vi "SPD.Set Meas Grid.vi"(8 "Error In":errorcluster, 9 "HV_GridParams":T1, 10 "SPD.DCR Meas Setup":T15={"Strobe_code"={"Start"=0.0, "Stop"=0.0, "Step"=0.0}, "Temperature"={"Start"=-45.0, "Stop"=-45.0, "Step"=2.5}} caption="Настройка Измерений", 11 "SPD.Stand Ctrl in":T2 {"spdDeviceSession"."hidSPD.Sturtup Values"."HV_bias" format="%#_6p, V"; "spdDeviceSession"."hidSPD.Sturtup Values"."TSet" format="%#_6p, DegC"; "spdDeviceSession"."hidSPD.Controller"."HV_bias" format="%#_6p, V"; "spdDeviceSession"."hidSPD.Controller"."TSet" format="%#_6p, DegC"}) -> (0 "Error Out":errorcluster, 3 "SPD.Stand Ctrl out":T2 {"spdDeviceSession"."hidSPD.Sturtup Values"."HV_bias" format="%#_6p, V"; "spdDeviceSession"."hidSPD.Sturtup Values"."TSet" format="%#_6p, DegC"; "spdDeviceSession"."hidSPD.Controller"."HV_bias" format="%#_6p, V"; "spdDeviceSession"."hidSPD.Controller"."TSet" format="%#_6p, DegC"})   [LabVIEW 2018]
uses:
  typedefs/SPD.Grid Meas Setup.ctl
  typedefs/SPD.Test Range.ctl
  typedefs/SPD.Stand Ctrl.ctl
  Instruments/SPD HID Interface/hidSPDLibForLabView/LibVIs/hidSPD Controls/hidSPD Device Session.ctl
  Instruments/SPD HID Interface/hidSPDLibForLabView/LibVIs/hidSPD Controls/hidSPD Controller.ctl
  Instruments/SPD HID Interface/hidSPDLibForLabView/LibVIs/hidSPD Controls/hidSPD SPD Type.ctl
  Instruments/KC705 DevBoard/typedefs/DevB.Session.ctl
  Instruments/KeySight 53230A/typedefs/FreqC.Session.ctl
  Instruments/KeySight 8164B/KeySight 8164B LAN InstrLib/typedefs/KeySight 8164B control.ctl
  Instruments/LeCroy SDA830/typedefs/LeCroy.Session.ctl
  typedefs/SPD.Events.ctl
  ConfigFile/SPD.Config File ctrl.ctl
  <vilib>/Utility/config.llb/Config Data RefNum.ctl
  typedefs/SPD.Meas Result.ctl
  typedefs/SPD.Queues.ctl
  typedefs/SPD.Stand state.ctl
  MeasGrid/typedefs/SPD.HV_Grid Test Params.ctl
  <vilib>/Analysis/1siggen.llb/Ramp Pattern by Delta.vi
  <vilib>/Analysis/NI_AALBase.lvlib
  Instruments/KeySight 8164B/KeySight 8164B LAN InstrLib.lvlib
  <vilib>/Utility/config.llb/NI_LVConfig.lvlib
  Instruments/SPD HID Interface/hidSPDLibForLabView/hidSPDLibForLabView.lvlib
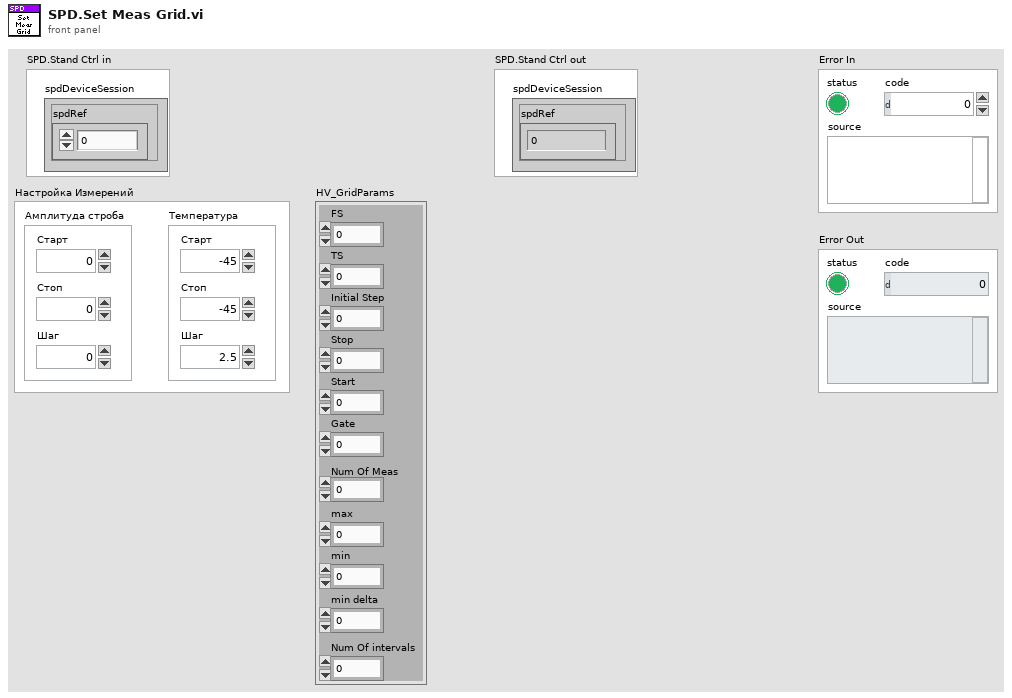
[diagram p1: front panel]
types:
  T1 = typedef "SPD.HV_Grid Test Params.ctl" = cluster{"FS":i32, "TS":i32, "Initial Step":dbl, "Stop":dbl, "Start":dbl, "Gate":dbl, "Num Of Meas":i32, "max":dbl, "min":dbl, "min delta":dbl, "Num Of intervals":i32}
  T2 = typedef "SPD.Stand Ctrl.ctl" = cluster{"spdDeviceSession":T3, "DevBSession":T6, "FreqCSession":T7, "8164BSession":T8, "LeCroySession":T9, "Events":T10, "configFile":T11, "SPD.Result":T13, "SPD.Queues":T14, "Console":refnum<vi>}
  T3 = typedef "hidSPDLibForLabView.lvlib/hidSPD Device Session.ctl" = cluster{"spdRef":u64, "connected":bool, "spdName":string, "hidSPD.Controller":T4, "hidSPD.Sturtup Values":T4, "SPD Type":T5}
  T4 = typedef "hidSPDLibForLabView.lvlib/hidSPD Controller.ctl" = cluster{"TSet":sgl, "HV_bias":sgl, "DDS_stb_code":u16}
  T5 = typedef "hidSPDLibForLabView.lvlib/hidSPD SPD Type.ctl" = enum16{"Free Run", "Gate"}
  T6 = typedef "DevB.Session.ctl" = cluster{"DevBRef":refnum<visa-resource-name>, "connected":bool}
  T7 = typedef "FreqC.Session.ctl" = cluster{"FreqCRef":refnum<visa-resource-name>, "timeout":dbl, "Gate":dbl, "connected":bool}
  T8 = typedef "KeySight 8164B LAN InstrLib.lvlib/KeySight 8164B control.ctl" = cluster{"Connection ID":refnum<k5>, "Connected":bool, "Info":string, "Slots Info":string[]}
  T9 = typedef "LeCroy.Session.ctl" = cluster{"LeCroySession":refnum<visa-resource-name>, "connected":bool}
  T10 = typedef "SPD.Events.ctl" = cluster{"DCRTest":refnum<user-event>, "Stop":refnum<user-event>}
  T11 = typedef "SPD.Config File ctrl.ctl" = cluster{"configFile ref":T12, "configFile path":path, "equipmentFile ref":T12}
  T12 = typedef "NI_LVConfig.lvlib/Config Data RefNum.ctl" = refnum<k1>
  T13 = typedef "SPD.Meas Result.ctl" = cluster{"HV_Bias":dbl[][][], "Stb_code":dbl[], "Temprature":dbl[], "Data":dbl[][][][], "DateTime":string}
  T14 = typedef "SPD.Queues.ctl" = cluster{"state queue":refnum<queue>}
  T15 = typedef "SPD.Grid Meas Setup.ctl" = cluster{"Strobe_code":T16, "Temperature":T16}
  T16 = typedef "SPD.Test Range.ctl" = cluster{"Start":dbl, "Stop":dbl, "Step":dbl}
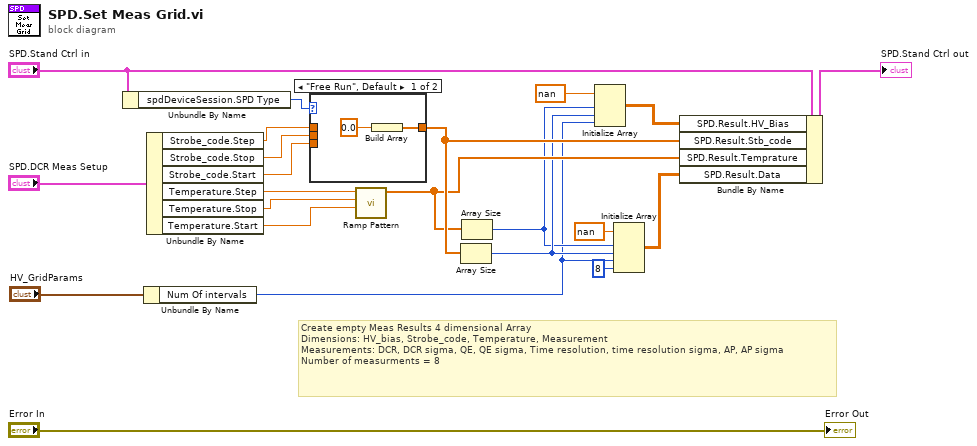
[diagram p0: block diagram]
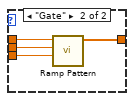
[diagram p2: hidden frame]
diagram:
  # "Create empty Meas Results 4 dimensional Array\nDimensions: HV_bias, Strobe_code, Temperature, Measurement\nMeasurements: DCR, DCR sigma, QE, QE sigma, Time resolution, time resolution sigma, AP, AP sigma\nNumber of measurments = 8"
  n1 = Unbundle By Name("SPD.Stand Ctrl in") -> ("spdDeviceSession.SPD Type"=w1:T5)
  n2 = Unbundle By Name("HV_GridParams") -> ("Num Of intervals"=w3:i32)
  n3 = Unbundle By Name("SPD.DCR Meas Setup") -> ("Strobe_code.Step"=w22:dbl, "Strobe_code.Stop"=w21:dbl, "Strobe_code.Start"=w20:dbl, "Temperature.Step"=w19:dbl, "Temperature.Stop"=w18:dbl, "Temperature.Start"=w17:dbl)
  n4 = case shown="\"Free Run\", Default" w1 {
    tunnel: w22 -> [_ w28]
    tunnel: w21 -> [_ w27]
    tunnel: w20 -> [_ w26]
    tunnel: [w23 w25] -> w12
    frame "Free Run", Default {
      n5 = Build Array(0.0) -> (w23:dbl[])
    }
    frame "Gate" {
      n6 = call-poly <vilib>:"Ramp Pattern.vi"("start"=w26, "end"=w27, "delta"=w28) -> ("Ramp Pattern"=w25:dbl[])  [unwired: 6 in, 2 out]
    }
  }
  n7 = call-poly <vilib>:"Ramp Pattern.vi"("start"=w17, "end"=w18, "delta"=w19) -> ("Ramp Pattern"=w11:dbl[])  [unwired: 6 in, 2 out]
  n8 = Array Size(array=w12) -> (size(s)=w7:i32)
  n9 = Array Size(array=w11) -> (size(s)=w4:i32)
  n10 = Initialize Array(nan ("element"), w4, w7, w3) -> (w5:dbl[][][])
  n11 = Initialize Array(nan ("element"), w4, w7, w3, 8 ("dimension size")) -> (w8:dbl[][][][])
  n12 = Bundle By Name(cluster="SPD.Stand Ctrl in", "SPD.Result.HV_Bias"=w5, "SPD.Result.Stb_code"=w12, "SPD.Result.Temprature"=w11, "SPD.Result.Data"=w8) -> (→"SPD.Stand Ctrl out":T2)
  "Error Out" <- "Error In"
